vi "Copper Mass Spec Control.vi"() -> ()   [LabVIEW 2021]
uses:
  <vilib>/LabVIEW Interface for Arduino/Type Defs/Pin Mode.ctl
  <vilib>/LabVIEW Interface for Arduino/LabVIEW Interface for Arduino.lvlib
panel:
  out "Power of chopper":bool
  in  "Chopper power on/off":bool
  out "error out":errorcluster
  in  "Stopp":bool
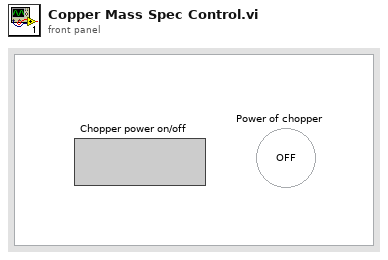
[diagram p1: front panel]
types:
  T1 = typedef "LabVIEW Interface for Arduino.lvlib/Pin Mode.ctl" = enum8{"Input", "Output"}
  T2 = typedef "LabVIEW Interface for Arduino.lvlib/Arduino Resource.ctl" = cluster{"VISA resource":refnum<visa-resource-name>, "Board Type":T3, "Connection Type":enum8{"USB / Serial"}, "Bytes Per Packet (15)":u8}
  T3 = typedef "LabVIEW Interface for Arduino.lvlib/Board Type.ctl" = enum16{"Uno", "Dimuelanove w/Atmega 328", "Mega 2560"}
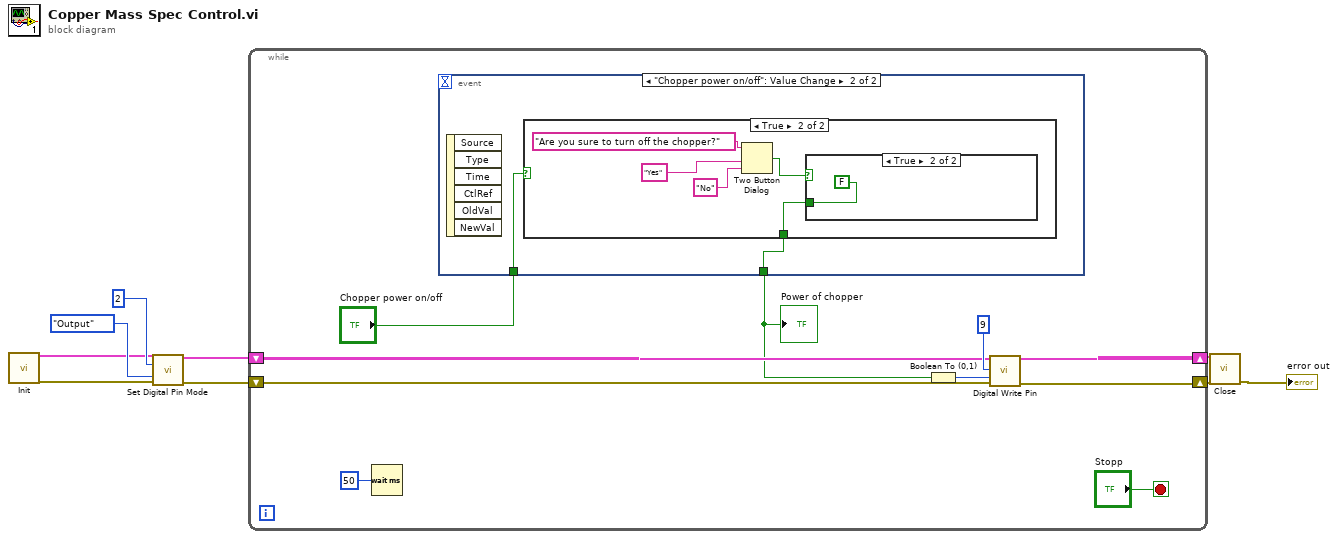
[diagram p0: block diagram]
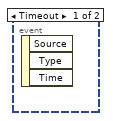
[diagram p2: hidden frame]
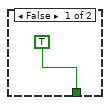
[diagram p3: hidden frame]
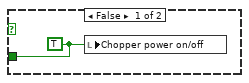
[diagram p4: hidden frame]
diagram:
  n1 = call <vilib>:"Init.vi"() -> ("Arduino Resource"=w3:T2, "error out"=w2:errorcluster)  [unwired: 18 in]
  n2 = call <vilib>:"Set Digital Pin Mode.vi"("Arduino Resource"=w3, "Digital I/O Pin"=u8 2, "Pin Mode (Input)"=Pin_Mode."Output", "error in"=w2) -> ("Arduino Resource"=w7:T2, "error out"=w6:errorcluster)  [unwired: 10 in]
  n3 = while {
    shift-right: [w13] -> w9
    shift-left: w7 -> [w15]
    shift-right: [w12] -> w8
    shift-left: w6 -> [w14]
    stop <- "Stopp" stop-if-true
    n4 = Wait (ms)(milliseconds to wait=u32 50 ("Zu wartende ms")) -> ()  [unwired: 1 out]
    n5 = event shown="[1] \"Chopper power on/off\": Value Change" {
      selector: _ -> [_ _]
      dyn-events: _ -> [_ _]
      timeout: _ -> [_ _]
      tunnel: [_ w21] -> w11
      tunnel: "Chopper power on/off" -> [_ w20]
      event Timeout {
        n6 = event-data() -> ()  [unwired: 1 in, 3 out]
      }
      event "Chopper power on/off": Value Change {
        n7 = event-data() -> ()  [unwired: 1 in, 6 out]
        n8 = case shown="True" w20 {
          tunnel: [TRUE ("T button?") w25] -> w21
          frame False {
          }
          frame True {
            n9 = Two Button Dialog(message="Are you sure to turn off the chopper?", 1:"No" ("F button name (\"Cancel\")"), 2:"Yes" ("T button name (\"OK\")")) -> (T button?=w26:bool)
            n10 = case shown="True" w26 {
              tunnel: [w28 FALSE] -> w25
              frame False {
                w28 = TRUE
                n11 = local write "Chopper power on/off"(w28) -> ()
              }
              frame True {
              }
            }
          }
        }
      }
    }
    "Power of chopper" <- w11
    n12 = Boolean To (0,1)(Boolean=w11) -> (0, 1=w16:i16)
    n13 = call <vilib>:"Digital Write Pin.vi"("Arduino Resource"=w15, "Digital I/O Pin (0)"=u8 9, "Value (0)"=w16, "error in"=w14) -> ("Arduino Resource"=w13:T2, "error out"=w12:errorcluster)  [unwired: 10 in]
  }
  n14 = call <vilib>:"Close.vi"("Arduino Resource"=w9, "error in"=w8) -> ("error out"=→"error out":errorcluster)  [unwired: 13 in]
